vi "Start Async Non-Reentrant.vi"(4 "Async Elements":refnum<queue>, 7 "Actor in":refnum<class "Actor.lvclass">, 8 "Error in":errorcluster) -> (0 "Error out":errorcluster)   [LabVIEW 2020, in "jettl.lvlib"]
uses:
  jettl.lvlib
  Msg/Msg.lvclass
  Transport/Transport.lvclass
  Actor/Actor.lvclass
  Actor.vi
  Actor Attributes.ctl
  Async Elements.ctl
  Msgs.ctl
  Msg Names.ctl
  Unified Layer.ctl
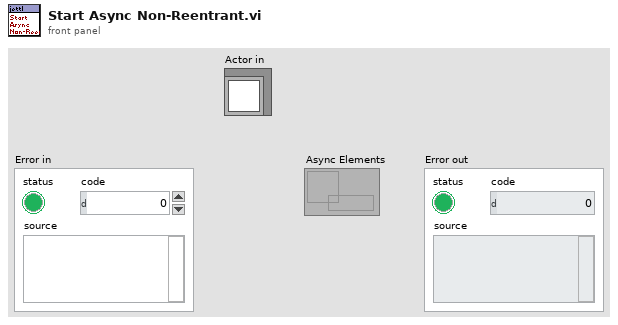
[diagram p1: front panel]
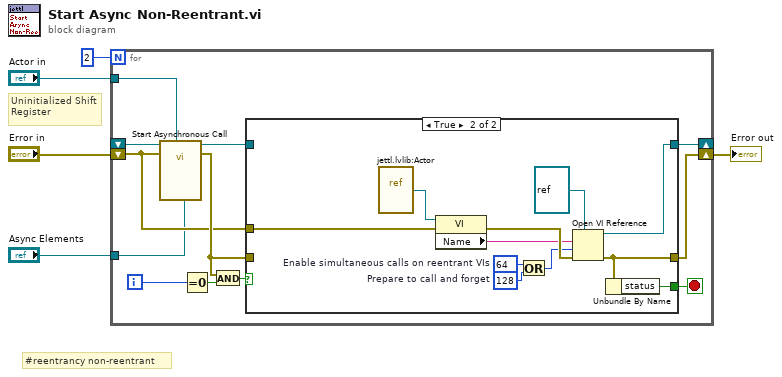
[diagram p0: block diagram]
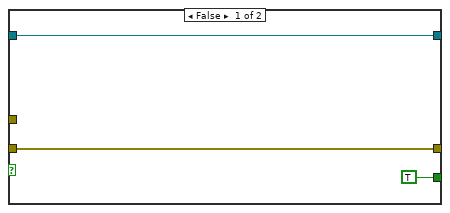
[diagram p2: hidden frame]
diagram:
  # "Uninitialized Shift Register"
  # "#reentrancy non-reentrant"
  n1 = for {
    N: 2 -> [_]
    shift-right: [w17] -> _
    shift-left: _ -> [w16]
    shift-right: [w14] -> w2
    shift-left: "Error in" -> [w8]
    tunnel: "Async Elements" -> [w6]
    tunnel: "Actor in" -> [w7]
    i -> [w11]
    stop <- w9 stop-if-true
    n2 = call-by-ref "Start Asynchronous Call"(reference=w16, error in=w8, "Async Elements"=w6, "Actor in"=w7) -> (reference out=w15:refnum<vi>, error out=w10:errorcluster)  [unwired: 8 in, 2 out]
    n3 = Equal To 0?(x=w11) -> (x = 0?=w12:bool)
    n4 = And(x=w10, y=w12) -> (x .and. y?=w13:bool)
    n5 = case shown="True" w13 {
      tunnel: [w20 w29] -> w17
      tunnel: [w19 w22] -> w14
      tunnel: w15 -> [w20 _]
      tunnel: w10 -> [w19 _]
      tunnel: [TRUE w21] -> w9
      tunnel: w8 -> [_ w28]
      frame False {
      }
      frame True {
        w24 = 64  # Enable simultaneous calls on reentrant VIs
        w25 = 128  # Prepare to call and forget
        n6 = vi-ref "jettl.lvlib:Actor.vi"() -> (w27:refnum<vi>)
        n7 = property class="VI"(reference=w27, error in=w28) -> (error out=w31:errorcluster, "Name"=w30:string)  [unwired: 1 out]
        n8 = Or(x=w24, y=w25) -> (x .or. y?=w23:i32)
        n9 = Open VI Reference(type specifier VI Refnum (for type only)=refnum<vi> refnum, vi path=w30, options=w23, error in (no error)=w31) -> (vi reference=w29:refnum<vi>, error out=w22:errorcluster)  [unwired: 2 in]
        n10 = Unbundle By Name(w22) -> ("status"=w21:bool)
      }
    }
  }
  "Error out" <- w2
